vi "Read Anything.vi"(7 "Type of Anything":variant, 8 "Error In":errorcluster, 9 "Section Name (Name of \"Type of Anything\")":string, 11 "Path (dialog)":path) -> (0 "Error Out":errorcluster, 1 "Found?":bool, 3 "Anything":variant)   [LabVIEW 2012]
doc: "This VI is designed to read data from a file written by <B>Write Anything.vi</B>. If the data type definition has changed since it was written to file, this VI will still read and fill out any elements of the cluster that have the same name. Any elements for which it cannot find a name match in the file will be supplied with their datatype's default value.\n\nFreeware from Moore Good Ideas, www.mooregoodideas.com. Do not remove this line."
uses:
  <vilib>/Utility/VariantDataType/VariantType.lvlib
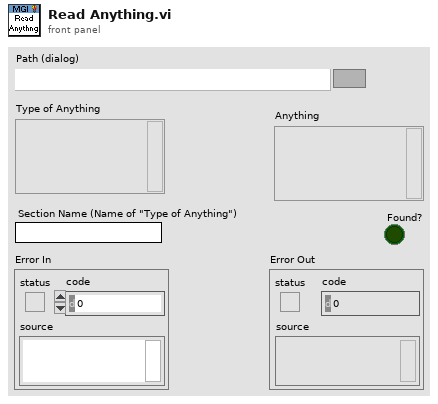
[diagram p1: front panel]
types:
  T1 = typedef "VariantType.lvlib/Type.ctl" = enum8{"Invalid Type", "Void", "I8", "I16", "I32", "I64", "U8", "U16", "U32", "U64", "Single Float", "Double Float", "Extended Float", "Single Complex", "Double Complex", "Extended Complex", "Enum U8", "Enum U16", "Enum U32", "Enum U64", "Single Float With Unit", "Double Float With Unit", "Extended Float With Unit", "Single Complex with Unit", "Double Complex with Unit", "Extended Complex with Unit", "Boolean", "String", "Path", "Picture", "Tag", "Array", "Cluster", "Variant", "LV Variant", "Waveform", "Timestamp", "Digital Waveform", "Digital Data", "ExpressData", "Refnum", "External Data", "VI", "Poly VI", "LabVIEW Class Instance", "Fixed Point"}
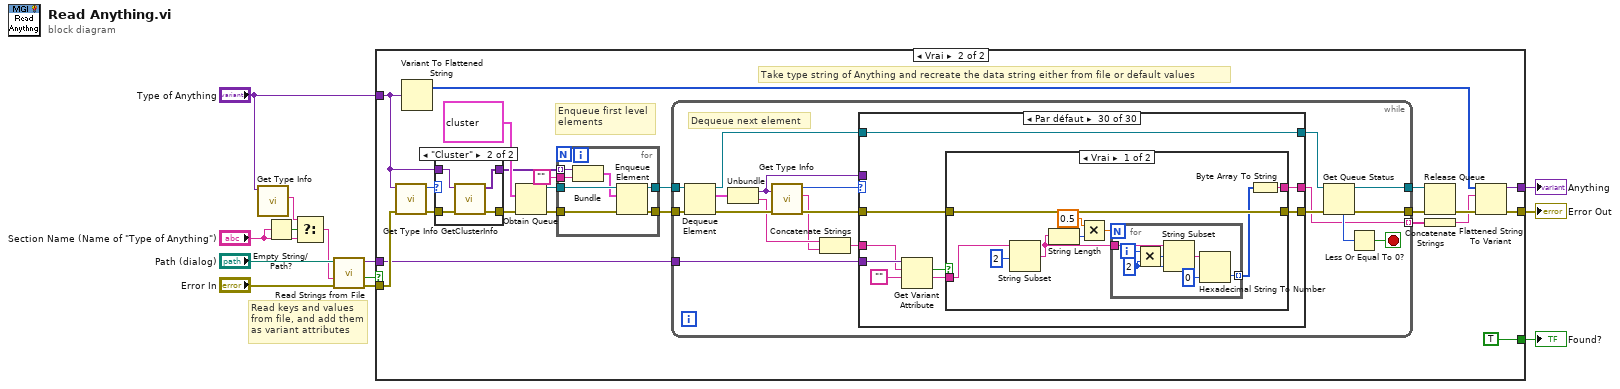
[diagram p0: block diagram]
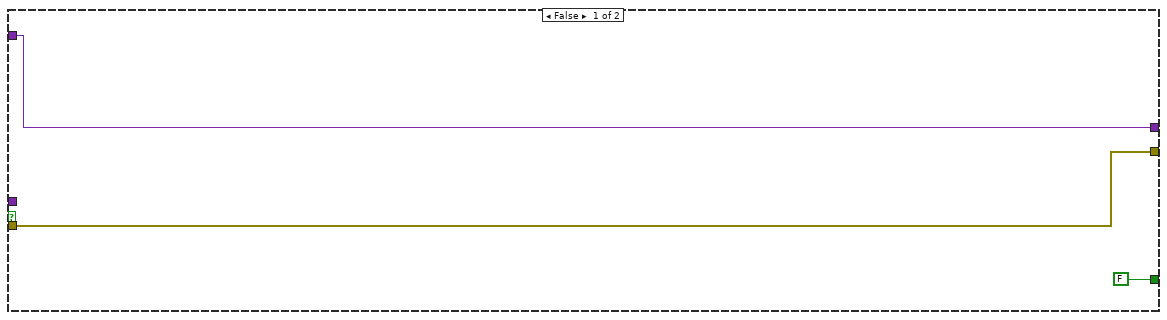
[diagram p2: hidden frame]
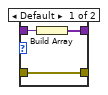
[diagram p3: hidden frame]
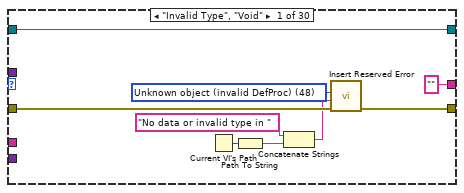
[diagram p4: hidden frame]
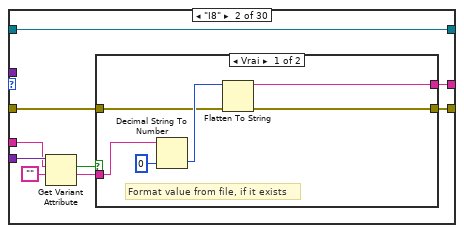
[diagram p5: hidden frame]
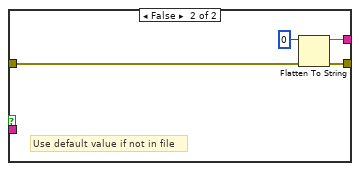
[diagram p6: hidden frame]
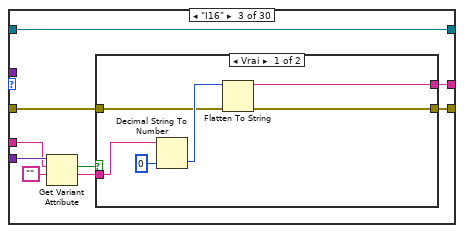
[diagram p7: hidden frame]
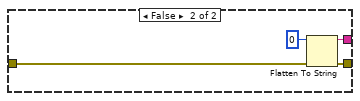
[diagram p8: hidden frame]
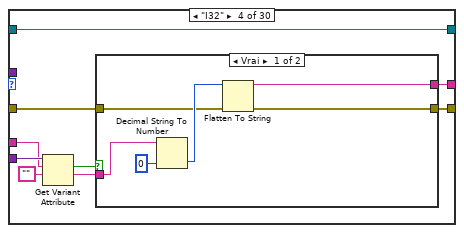
[diagram p9: hidden frame]
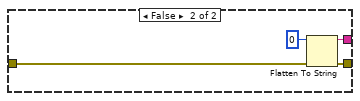
[diagram p10: hidden frame]
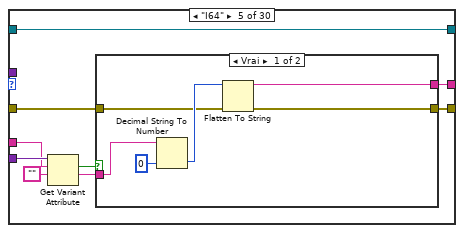
[diagram p11: hidden frame]
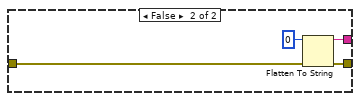
[diagram p12: hidden frame]
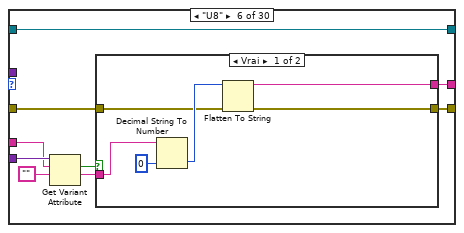
[diagram p13: hidden frame]
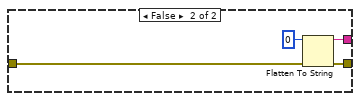
[diagram p14: hidden frame]
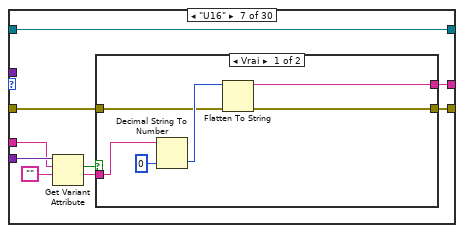
[diagram p15: hidden frame]
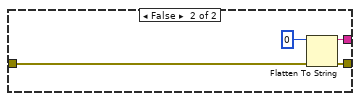
[diagram p16: hidden frame]
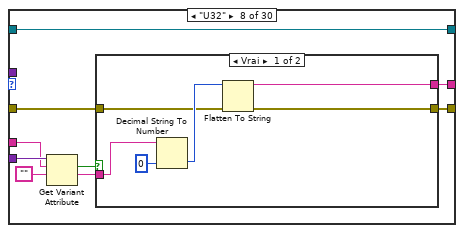
[diagram p17: hidden frame]
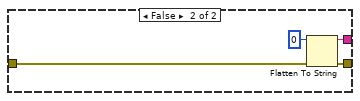
[diagram p18: hidden frame]
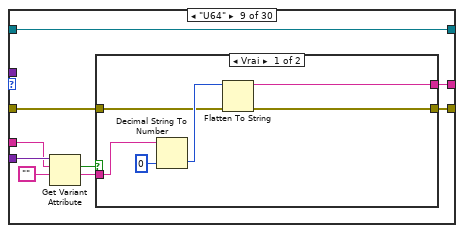
[diagram p19: hidden frame]
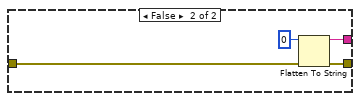
[diagram p20: hidden frame]
diagram:
  # "Read keys and values from file, and add them as variant attributes"
  n1 = call "Get Type Info.vi"("Variant"="Type of Anything") -> ("Name"=w2:string)  [unwired: 8 in, 2 out]
  n2 = Empty String/Path?(string/path="Section Name (Name of \"Type of Anything\")") -> (empty?=w5:bool)
  n3 = Select(t=w2, s=w5, f="Section Name (Name of \"Type of Anything\")") -> (s? t:f=w3:string)
  n4 = call "Read Strings from File.vi"("Error In"="Error In", "Section Name"=w3, "Path"="Path (dialog)") -> ("Error Out"=w11:errorcluster, "Found?"=w8:bool, "Variant Database"=w7:variant)  [unwired: 6 in]
  n5 = case shown="Vrai" w8 {
    tunnel: [w15 w37] -> w13
    tunnel: [w16 w36] -> w12
    tunnel: "Type of Anything" -> [w16 w18]
    tunnel: w11 -> [w15 w24]
    tunnel: [FALSE TRUE] -> w9
    tunnel: w7 -> [_ w22]
    frame False {
    }
    frame True {
      # "Enqueue first level\nelements"
      # "Take type string of Anything and recreate the data string either from file or default values"
      n6 = call "Get Type Info.vi"("Error In"=w24, "Variant"=w18) -> ("Error Out"=w19:errorcluster, "Type Enum"=w21:T1)  [unwired: 7 in, 1 out]
      n7 = Variant To Flattened String(Variant=w18) -> (1:w38:i16[])  [unwired: 1 out]
      n8 = case shown="\"Cluster\"" w21 {
        tunnel: [w41 w44] -> w20
        tunnel: w19 -> [w41 w45]
        tunnel: w18 -> [w40 w43]
        tunnel: [w39 w42] -> w17
        frame Default {
          n9 = Build Array(w40) -> (w39:variant[])
        }
        frame "Cluster" {
          n10 = call <vilib>:"GetClusterInfo.vi"("error in (no error)"=w45, "Variant"=w43) -> ("error out"=w44:errorcluster, "Cluster Elements"=w42:variant[])  [unwired: 8 in]
        }
      }
      n11 = Obtain Queue(element data type=cluster{"Variant":variant, "Name":string} {"Variant"=variant, "Name"=""}, error in (no error)=w20) -> (queue out=w34:refnum<queue>, error out=w26:errorcluster)  [unwired: 3 in, 1 out]
      n12 = for {
        tunnel: w34 -> [w52]
        tunnel: [w51] -> w33
        tunnel: [w50] -> w32
        tunnel: w17 -> [w49] mode=indexing
        tunnel: "" -> [w47]
        tunnel: w26 -> [w46]
        n13 = Bundle("ArrayElt"=w49, w47) -> (w48:cluster{"ArrayElt":variant, string})  [unwired: 1 in]
        n14 = Enqueue Element(queue=w52, element=w48, error in (no error)=w46) -> (queue out=w50:refnum<queue>, error out=w51:errorcluster)  [unwired: 1 in, 1 out]
      }
      n15 = while {
        tunnel: w33 -> [w69]
        tunnel: [w64] -> w31
        tunnel: w22 -> [w56]
        tunnel: [w53] -> w35 mode=indexing
        tunnel: w32 -> [w66]
        tunnel: [w60] -> w29
        stop <- w61 stop-if-true
        # "Dequeue next element"
        n16 = Dequeue Element(queue=w66, error in (no error)=w69) -> (queue out=w67:refnum<queue>, element=w59:cluster{"Variant":variant, "Name":string}, error out=w68:errorcluster)  [unwired: 1 in, 1 out]
        n17 = Unbundle(w59) -> ("Variant"=w55:variant, "Name"=w57:string)
        n18 = call "Get Type Info.vi"("Error In"=w68, "Variant"=w55) -> ("Error Out"=w70:errorcluster, "Name"=w54:string, "Type Enum"=w71:T1)  [unwired: 7 in]
        n19 = Concatenate Strings(w57, w54) -> (w58:string)
        n20 = case shown="Par défaut" w71 {
          tunnel: [w74 w89 w108 w127 w146 w165 w184 w203 w222 w241 w261 w281 w301 w320 w339 w359 w385 w411 w437 w462 w481 w498 w513 w535 w564 w593 w622 w651 w679 w691] -> w65
          tunnel: w70 -> [w75 w88 w107 w126 w145 w164 w183 w202 w221 w240 w260 w280 w300 w319 w338 w358 w384 w410 w436 w461 w480 w497 w519 w534 w563 w592 w621 w650 w680 w690]
          tunnel: w58 -> [_ w83 w102 w121 w140 w159 w177 w197 w216 w235 w254 w275 w294 w314 w334 w351 w377 w404 w430 w456 w475 w491 w509 w529 w558 w586 w614 w644 w674 w683]
          tunnel: ["" ("data string") w87 w106 w125 w144 w163 w182 w201 w220 w239 w259 w279 w299 w318 w337 w357 w383 w409 w435 w460 w479 w496 "" w533 w562 w591 w620 w649 w677 w689] -> w53
          tunnel: w55 -> [_ _ _ _ _ _ _ _ _ _ _ _ _ _ _ w356 w382 w408 w434 _ _ _ w518 _ _ _ _ _ w678 _]
          tunnel: w67 -> [w76 w86 w105 w124 w143 w162 w181 w200 w219 w238 w258 w278 w298 w317 w336 w355 w381 w407 w433 w459 w478 w495 w514 w532 w561 w590 w619 w648 w682 w688]
          tunnel: [w76 w86 w105 w124 w143 w162 w181 w200 w219 w238 w258 w278 w298 w317 w336 w355 w381 w407 w433 w459 w478 w495 w512 w532 w561 w590 w619 w648 w681 w688] -> w63
          tunnel: w56 -> [_ w84 w103 w122 w141 w160 w178 w198 w217 w237 w255 w276 w295 w315 w335 w353 w378 w405 w431 w457 w476 w492 _ w530 w559 w588 w617 w645 w675 w686]
          frame "Invalid Type", "Void" {
            w72 = u16 48 items=["No error", "Argument error", "Memory is full", "Out of zone", "End of file", "File already open", "Generic file I/O error", "File not found", "File permission error", "Disk is full", "Duplicate path", "Too many files open", "System feature not enabled", "Resource file not found", "Cannot add resource", "Resource not found", "Image not found", "Image memory error", "Pen does not exist", "Config type invalid", "Config token not found", "Config parse error", "Config memory error", "Bad external code format", "Bad external code offset", "External code not present", "Null window", "Destroy window error", "Null menu", "Print aborted", "Bad print record", "Print driver error", "Windows error during printing", "Memory error during printing", "Print dialog error", "Generic print error", "Invalid device refnum", "Device not found", "Device parameter error", "Device unit error", "Cannot open device", "Device call aborted", "Generic error", "Cancelled by user", "Object ID too low", "Object ID too high", "Object not in heap", "Unknown heap", "Unknown object (invalid DefProc)", "Unknown object (DefProc not in table)", "Message out of range", "Invalid (null) method", "Unknown message", "Manager call not supported", "Bad address", "Network operation in progress", "Network operation timed out", "Connection is busy", "Network attribute not supported", "Network error", "Address in use", "System out of memory", "Connection aborted", "Connection refused", "Not connected", "Already connected", "Connection closed", "Initialization error (interapplication manager)", "Bad occurrence", "Wait on unbound occurrence handler", "Occurrence queue overflow", "Datalog type conflict", "Unused", "Unrecognized type (interapplication manager)", "Memory corrupt", "Failed to make temporary DLL", "Old CIN version", "Drag socket not found", "Failed to load drop-object", "Failed to register OLE object", "Failed to release OLE object", "Format specifier type mismatch", "Unknown format specifier", "Too few format specifiers", "Too many format specifiers", "Scan failed", "Newer CIN version", "OLE Convert", "Runtime menu error", "Password tampered", "Unknown error code"] ("Reserved Error Code")
            n21 = Current VI's Path() -> (path=w78:path)
            n22 = Path To String(path=w78) -> (string=w77:string)
            n23 = Concatenate Strings("No data or invalid type in " ("string"), w77) -> (w73:string)
            n24 = call "Insert Reserved Error.vi"("error in (no error)"=w75, "non-standard source (\"\")"=w73, "Reserved Error Code"=w72) -> ("error out"=w74:errorcluster)  [unwired: 4 in]
          }
          frame "I8" {
            n25 = Get Variant Attribute(Variant=w84, name=w83, default value (empty Variant)="") -> (found=w81:bool, value=w82:string)  [unwired: 1 in, 2 out]
            n26 = case shown="Vrai" w81 {
              tunnel: w82 -> [w90 _]
              tunnel: [w93 w96] -> w89
              tunnel: w88 -> [w92 w97]
              tunnel: [w94 w99] -> w87
              frame True {
                # "Format value from file, if it exists"
                n27 = Decimal String To Number(string=w90, default (0L)=i8 0 ("default (0 I32)")) -> (number=w95:i8)  [unwired: 1 in, 1 out]
                n28 = Flatten To String(anything=w95, error in (no error)=w92) -> (data string=w94:string, error out=w93:errorcluster)  [unwired: 2 in, 1 out]
              }
              frame False {
                # "Use default value if not in file"
                n29 = Flatten To String(anything=i8 0, error in (no error)=w97) -> (data string=w99:string, error out=w96:errorcluster)  [unwired: 2 in, 1 out]
              }
            }
          }
          frame "I16" {
            n30 = Get Variant Attribute(Variant=w103, name=w102, default value (empty Variant)="") -> (found=w100:bool, value=w101:string)  [unwired: 1 in, 2 out]
            n31 = case shown="Vrai" w100 {
              tunnel: w101 -> [w109 _]
              tunnel: [w112 w115] -> w108
              tunnel: w107 -> [w111 w116]
              tunnel: [w113 w118] -> w106
              frame True {
                n32 = Decimal String To Number(string=w109, default (0L)=i16 0 ("default (0 I32)")) -> (number=w114:i16)  [unwired: 1 in, 1 out]
                n33 = Flatten To String(anything=w114, error in (no error)=w111) -> (data string=w113:string, error out=w112:errorcluster)  [unwired: 2 in, 1 out]
              }
              frame False {
                n34 = Flatten To String(anything=i16 0, error in (no error)=w116) -> (data string=w118:string, error out=w115:errorcluster)  [unwired: 2 in, 1 out]
              }
            }
          }
          frame "I32" {
            n35 = Get Variant Attribute(Variant=w122, name=w121, default value (empty Variant)="") -> (found=w119:bool, value=w120:string)  [unwired: 1 in, 2 out]
            n36 = case shown="Vrai" w119 {
              tunnel: w120 -> [w128 _]
              tunnel: [w131 w134] -> w127
              tunnel: w126 -> [w130 w135]
              tunnel: [w132 w137] -> w125
              frame True {
                n37 = Decimal String To Number(string=w128, default (0L)=0 ("default (0 I32)")) -> (number=w133:i32)  [unwired: 1 in, 1 out]
                n38 = Flatten To String(anything=w133, error in (no error)=w130) -> (data string=w132:string, error out=w131:errorcluster)  [unwired: 2 in, 1 out]
              }
              frame False {
                n39 = Flatten To String(anything=0, error in (no error)=w135) -> (data string=w137:string, error out=w134:errorcluster)  [unwired: 2 in, 1 out]
              }
            }
          }
          frame "I64" {
            n40 = Get Variant Attribute(Variant=w141, name=w140, default value (empty Variant)="") -> (found=w138:bool, value=w139:string)  [unwired: 1 in, 2 out]
            n41 = case shown="Vrai" w138 {
              tunnel: w139 -> [w147 _]
              tunnel: [w150 w153] -> w146
              tunnel: w145 -> [w149 w154]
              tunnel: [w151 w156] -> w144
              frame True {
                n42 = Decimal String To Number(string=w147, default (0L)=i64 0 ("default (0 I32)")) -> (number=w152:i64)  [unwired: 1 in, 1 out]
                n43 = Flatten To String(anything=w152, error in (no error)=w149) -> (data string=w151:string, error out=w150:errorcluster)  [unwired: 2 in, 1 out]
              }
              frame False {
                n44 = Flatten To String(anything=i64 0, error in (no error)=w154) -> (data string=w156:string, error out=w153:errorcluster)  [unwired: 2 in, 1 out]
              }
            }
          }
          frame "U8" {
            n45 = Get Variant Attribute(Variant=w160, name=w159, default value (empty Variant)="") -> (found=w157:bool, value=w158:string)  [unwired: 1 in, 2 out]
            n46 = case shown="Vrai" w157 {
              tunnel: w158 -> [w166 _]
              tunnel: [w169 w172] -> w165
              tunnel: w164 -> [w168 w173]
              tunnel: [w170 w175] -> w163
              frame True {
                n47 = Decimal String To Number(string=w166, default (0L)=u8 0 ("default (0 I32)")) -> (number=w171:u8)  [unwired: 1 in, 1 out]
                n48 = Flatten To String(anything=w171, error in (no error)=w168) -> (data string=w170:string, error out=w169:errorcluster)  [unwired: 2 in, 1 out]
              }
              frame False {
                n49 = Flatten To String(anything=u8 0, error in (no error)=w173) -> (data string=w175:string, error out=w172:errorcluster)  [unwired: 2 in, 1 out]
              }
            }
          }
          frame "U16" {
            n50 = Get Variant Attribute(Variant=w178, name=w177, default value (empty Variant)="") -> (found=w176:bool, value=w179:string)  [unwired: 1 in, 2 out]
            n51 = case shown="Vrai" w176 {
              tunnel: w179 -> [w185 _]
              tunnel: [w188 w191] -> w184
              tunnel: w183 -> [w187 w192]
              tunnel: [w189 w194] -> w182
              frame True {
                n52 = Decimal String To Number(string=w185, default (0L)=u16 0 ("default (0 I32)")) -> (number=w190:u16)  [unwired: 1 in, 1 out]
                n53 = Flatten To String(anything=w190, error in (no error)=w187) -> (data string=w189:string, error out=w188:errorcluster)  [unwired: 2 in, 1 out]
              }
              frame False {
                n54 = Flatten To String(anything=u16 0, error in (no error)=w192) -> (data string=w194:string, error out=w191:errorcluster)  [unwired: 2 in, 1 out]
              }
            }
          }
          frame "U32" {
            n55 = Get Variant Attribute(Variant=w198, name=w197, default value (empty Variant)="") -> (found=w195:bool, value=w196:string)  [unwired: 1 in, 2 out]
            n56 = case shown="Vrai" w195 {
              tunnel: w196 -> [w204 _]
              tunnel: [w207 w210] -> w203
              tunnel: w202 -> [w206 w211]
              tunnel: [w208 w213] -> w201
              frame True {
                n57 = Decimal String To Number(string=w204, default (0L)=u32 0 ("default (0 I32)")) -> (number=w209:u32)  [unwired: 1 in, 1 out]
                n58 = Flatten To String(anything=w209, error in (no error)=w206) -> (data string=w208:string, error out=w207:errorcluster)  [unwired: 2 in, 1 out]
              }
              frame False {
                n59 = Flatten To String(anything=u32 0, error in (no error)=w211) -> (data string=w213:string, error out=w210:errorcluster)  [unwired: 2 in, 1 out]
              }
            }
          }
          frame "U64" {
            n60 = Get Variant Attribute(Variant=w217, name=w216, default value (empty Variant)="") -> (found=w214:bool, value=w215:string)  [unwired: 1 in, 2 out]
            n61 = case shown="Vrai" w214 {
              tunnel: w215 -> [w223 _]
              tunnel: [w226 w229] -> w222
              tunnel: w221 -> [w225 w230]
              tunnel: [w227 w232] -> w220
              frame True {
                n62 = Decimal String To Number(string=w223, default (0L)=u64 0 ("default (0 I32)")) -> (number=w228:u64)  [unwired: 1 in, 1 out]
                n63 = Flatten To String(anything=w228, error in (no error)=w225) -> (data string=w227:string, error out=w226:errorcluster)  [unwired: 2 in, 1 out]
              }
              frame False {
                n64 = Flatten To String(anything=u64 0, error in (no error)=w230) -> (data string=w232:string, error out=w229:errorcluster)  [unwired: 2 in, 1 out]
              }
            }
          }
          frame "Single Float", "Single Float With Unit" {
            n65 = Get Variant Attribute(Variant=w237, name=w235, default value (empty Variant)="") -> (found=w233:bool, value=w234:string)  [unwired: 1 in, 2 out]
            n66 = case shown="Vrai" w233 {
              tunnel: w234 -> [w243 _]
              tunnel: [w246 w249] -> w241
              tunnel: w240 -> [w245 w250]
              tunnel: [w247 w252] -> w239
              frame True {
                n67 = Fract/Exp String To Number(use system decimal point (T)=FALSE ("utiliser le séparateur décimal du système (V)"), string=w243, default (0 dbl)=sgl 0.0 ("default (0 I32)")) -> (number=w248:sgl)  [unwired: 1 in, 1 out]
                n68 = Flatten To String(anything=w248, error in (no error)=w245) -> (data string=w247:string, error out=w246:errorcluster)  [unwired: 2 in, 1 out]
              }
              frame False {
                n69 = Flatten To String(anything=sgl 0.0, error in (no error)=w250) -> (data string=w252:string, error out=w249:errorcluster)  [unwired: 2 in, 1 out]
              }
            }
          }
          frame "Double Float", "Double Float With Unit" {
            n70 = Get Variant Attribute(Variant=w255, name=w254, default value (empty Variant)="") -> (found=w253:bool, value=w256:string)  [unwired: 1 in, 2 out]
            n71 = case shown="Vrai" w253 {
              tunnel: w256 -> [w263 _]
              tunnel: [w266 w269] -> w261
              tunnel: w260 -> [w265 w270]
              tunnel: [w267 w272] -> w259
              frame True {
                n72 = Fract/Exp String To Number(use system decimal point (T)=FALSE ("utiliser le séparateur décimal du système (V)"), string=w263, default (0 dbl)=0.0 ("default (0 DBL)")) -> (number=w268:dbl)  [unwired: 1 in, 1 out]
                n73 = Flatten To String(anything=w268, error in (no error)=w265) -> (data string=w267:string, error out=w266:errorcluster)  [unwired: 2 in, 1 out]
              }
              frame False {
                n74 = Flatten To String(anything=0.0, error in (no error)=w270) -> (data string=w272:string, error out=w269:errorcluster)  [unwired: 2 in, 1 out]
              }
            }
          }
          frame "Extended Float", "Extended Float With Unit" {
            n75 = Get Variant Attribute(Variant=w276, name=w275, default value (empty Variant)="") -> (found=w273:bool, value=w274:string)  [unwired: 1 in, 2 out]
            n76 = case shown="Vrai" w273 {
              tunnel: w274 -> [w283 _]
              tunnel: [w286 w289] -> w281
              tunnel: w280 -> [w285 w290]
              tunnel: [w287 w292] -> w279
              frame True {
                n77 = Fract/Exp String To Number(use system decimal point (T)=FALSE ("utiliser le séparateur décimal du système (V)"), string=w283, default (0 dbl)=ext 0.0 ("default (0 DBL)")) -> (number=w288:ext)  [unwired: 1 in, 1 out]
                n78 = Flatten To String(anything=w288, error in (no error)=w285) -> (data string=w287:string, error out=w286:errorcluster)  [unwired: 2 in, 1 out]
              }
              frame False {
                n79 = Flatten To String(anything=ext 0.0, error in (no error)=w290) -> (data string=w292:string, error out=w289:errorcluster)  [unwired: 2 in, 1 out]
              }
            }
          }
          frame "Single Complex", "Single Complex with Unit" {
            n80 = Get Variant Attribute(Variant=w295, name=w294, default value (empty Variant)="") -> (found=w293:bool, value=w296:string)  [unwired: 1 in, 2 out]
            n81 = case shown="Vrai" w293 {
              tunnel: w296 -> [w302 _]
              tunnel: [w306 w308] -> w301
              tunnel: w300 -> [w305 w309]
              tunnel: [w307 w311] -> w299
              frame True {
                n82 = Scan From String(input string=w302, default 1=csg 0.0+0.0i ("default (0 DBL)")) -> (output 1=w303:csg)  [unwired: 3 in, 3 out]
                n83 = Flatten To String(anything=w303, error in (no error)=w305) -> (data string=w307:string, error out=w306:errorcluster)  [unwired: 2 in, 1 out]
              }
              frame False {
                n84 = Flatten To String(anything=csg 0.0+0.0i, error in (no error)=w309) -> (data string=w311:string, error out=w308:errorcluster)  [unwired: 2 in, 1 out]
              }
            }
          }
          frame "Double Complex", "Double Complex with Unit" {
            n85 = Get Variant Attribute(Variant=w315, name=w314, default value (empty Variant)="") -> (found=w312:bool, value=w313:string)  [unwired: 1 in, 2 out]
            n86 = case shown="Vrai" w312 {
              tunnel: w313 -> [w321 _]
              tunnel: [w325 w327] -> w320
              tunnel: w319 -> [w324 w328]
              tunnel: [w326 w330] -> w318
              frame True {
                n87 = Scan From String(input string=w321, default 1=cdb 0.0+0.0i ("default (0 DBL)")) -> (output 1=w323:cdb)  [unwired: 3 in, 3 out]
                n88 = Flatten To String(anything=w323, error in (no error)=w324) -> (data string=w326:string, error out=w325:errorcluster)  [unwired: 2 in, 1 out]
              }
              frame False {
                n89 = Flatten To String(anything=cdb 0.0+0.0i, error in (no error)=w328) -> (data string=w330:string, error out=w327:errorcluster)  [unwired: 2 in, 1 out]
              }
            }
          }
          frame "Extended Complex", "Extended Complex with Unit" {
            n90 = Get Variant Attribute(Variant=w335, name=w334, default value (empty Variant)="") -> (found=w331:bool, value=w332:string)  [unwired: 1 in, 2 out]
            n91 = case shown="Vrai" w331 {
              tunnel: w332 -> [w340 _]
              tunnel: [w344 w346] -> w339
              tunnel: w338 -> [w343 w347]
              tunnel: [w345 w349] -> w337
              frame True {
                n92 = Scan From String(input string=w340, default 1=cxt 0.0+0.0i ("default (0 DBL)")) -> (output 1=w341:cxt)  [unwired: 3 in, 3 out]
                n93 = Flatten To String(anything=w341, error in (no error)=w343) -> (data string=w345:string, error out=w344:errorcluster)  [unwired: 2 in, 1 out]
              }
              frame False {
                n94 = Flatten To String(anything=cxt 0.0+0.0i, error in (no error)=w347) -> (data string=w349:string, error out=w346:errorcluster)  [unwired: 2 in, 1 out]
              }
            }
          }
          frame "Enum U8" {
            n95 = Get Variant Attribute(Variant=w353, name=w351, default value (empty Variant)="") -> (found=w350:bool, value=w352:string)  [unwired: 1 in, 2 out]
            n96 = case shown="Vrai" w350 {
              tunnel: w352 -> [w360 _]
              tunnel: [w370 w373] -> w359
              tunnel: w358 -> [w369 w374]
              tunnel: [w371 w375] -> w357
              tunnel: w356 -> [w368 _]
              frame True {
                n97 = call <vilib>:"GetNumericInfo.vi"("error in (no error)"=w369, "Variant"=w368) -> ("error out"=w361:errorcluster, "EnumNames"=w367:string[])  [unwired: 6 in, 2 out]
                n98 = Search 1D Array(1D array=w367, element=w360) -> (index of element=w366:i32)  [unwired: 1 in]
                n99 = In Range and Coerce(upper limit=255, x=w366, lower limit=0) -> (coerced(x)=w364:i32)  [unwired: 1 out]
                n100 = To Unsigned Byte Integer(number=w364) -> (unsigned 8bit integer=w365:u8)
                n101 = Flatten To String(anything=w365, error in (no error)=w361) -> (data string=w371:string, error out=w370:errorcluster)  [unwired: 2 in, 1 out]
              }
              frame False {
                n102 = Flatten To String(anything=u8 0, error in (no error)=w374) -> (data string=w375:string, error out=w373:errorcluster)  [unwired: 2 in, 1 out]
              }
            }
          }
          frame "Enum U16" {
            n103 = Get Variant Attribute(Variant=w378, name=w377, default value (empty Variant)="") -> (found=w376:bool, value=w379:string)  [unwired: 1 in, 2 out]
            n104 = case shown="Vrai" w376 {
              tunnel: w379 -> [w386 _]
              tunnel: [w396 w399] -> w385
              tunnel: w384 -> [w395 w400]
              tunnel: [w397 w401] -> w383
              tunnel: w382 -> [w394 _]
              frame True {
                n105 = call <vilib>:"GetNumericInfo.vi"("error in (no error)"=w395, "Variant"=w394) -> ("error out"=w387:errorcluster, "EnumNames"=w393:string[])  [unwired: 6 in, 2 out]
                n106 = Search 1D Array(1D array=w393, element=w386) -> (index of element=w392:i32)  [unwired: 1 in]
                n107 = In Range and Coerce(upper limit=u16 65535, x=w392, lower limit=0) -> (coerced(x)=w390:i32)  [unwired: 1 out]
                n108 = To Unsigned Word Integer(number=w390) -> (unsigned 16bit integer=w391:u16)
                n109 = Flatten To String(anything=w391, error in (no error)=w387) -> (data string=w397:string, error out=w396:errorcluster)  [unwired: 2 in, 1 out]
              }
              frame False {
                n110 = Flatten To String(anything=u16 0, error in (no error)=w400) -> (data string=w401:string, error out=w399:errorcluster)  [unwired: 2 in, 1 out]
              }
            }
          }
          frame "Enum U32" {
            n111 = Get Variant Attribute(Variant=w405, name=w404, default value (empty Variant)="") -> (found=w402:bool, value=w403:string)  [unwired: 1 in, 2 out]
            n112 = case shown="Vrai" w402 {
              tunnel: w403 -> [w412 _]
              tunnel: [w422 w425] -> w411
              tunnel: w410 -> [w421 w426]
              tunnel: [w423 w427] -> w409
              tunnel: w408 -> [w420 _]
              frame True {
                n113 = call <vilib>:"GetNumericInfo.vi"("error in (no error)"=w421, "Variant"=w420) -> ("error out"=w413:errorcluster, "EnumNames"=w419:string[])  [unwired: 6 in, 2 out]
                n114 = Search 1D Array(1D array=w419, element=w412) -> (index of element=w418:i32)  [unwired: 1 in]
                n115 = In Range and Coerce(upper limit=u32 4294967295, x=w418, lower limit=0) -> (coerced(x)=w416:u32)  [unwired: 1 out]
                n116 = To Unsigned Long Integer(number=w416) -> (unsigned 32bit integer=w417:u32)
                n117 = Flatten To String(anything=w417, error in (no error)=w413) -> (data string=w423:string, error out=w422:errorcluster)  [unwired: 2 in, 1 out]
              }
              frame False {
                n118 = Flatten To String(anything=u32 0, error in (no error)=w426) -> (data string=w427:string, error out=w425:errorcluster)  [unwired: 2 in, 1 out]
              }
            }
          }
          frame "Enum U64" {
            n119 = Get Variant Attribute(Variant=w431, name=w430, default value (empty Variant)="") -> (found=w428:bool, value=w429:string)  [unwired: 1 in, 2 out]
            n120 = case shown="Vrai" w428 {
              tunnel: [w448 w451] -> w437
              tunnel: w436 -> [w447 w452]
              tunnel: [w449 w453] -> w435
              tunnel: w434 -> [w446 _]
              tunnel: w429 -> [w438 _]
              frame True {
                n121 = call <vilib>:"GetNumericInfo.vi"("error in (no error)"=w447, "Variant"=w446) -> ("error out"=w439:errorcluster, "EnumNames"=w445:string[])  [unwired: 6 in, 2 out]
                n122 = Search 1D Array(1D array=w445, element=w438) -> (index of element=w444:i32)  [unwired: 1 in]
                n123 = In Range and Coerce(upper limit=u64 18446744073709551615, x=w444, lower limit=0) -> (coerced(x)=w442:u64)  [unwired: 1 out]
                n124 = To Unsigned Quad Integer(1:w442) -> (0:w443:u64)
                n125 = Flatten To String(anything=w443, error in (no error)=w439) -> (data string=w449:string, error out=w448:errorcluster)  [unwired: 2 in, 1 out]
              }
              frame False {
                n126 = Flatten To String(anything=u64 0, error in (no error)=w452) -> (data string=w453:string, error out=w451:errorcluster)  [unwired: 2 in, 1 out]
              }
            }
          }
          frame "Boolean" {
            n127 = Get Variant Attribute(Variant=w457, name=w456, default value (empty Variant)="") -> (found=w454:bool, value=w455:string)  [unwired: 1 in, 2 out]
            n128 = case shown="Vrai" w454 {
              tunnel: w455 -> [w463 _]
              tunnel: [w467 w470] -> w462
              tunnel: w461 -> [w464 w471]
              tunnel: [w468 w472] -> w460
              frame True {
                n129 = Equal?(x=w463, y="TRUE") -> (x = y?=w465:bool)
                n130 = Flatten To String(anything=w465, error in (no error)=w464) -> (data string=w468:string, error out=w467:errorcluster)  [unwired: 2 in, 1 out]
              }
              frame False {
                n131 = Flatten To String(anything=FALSE, error in (no error)=w471) -> (data string=w472:string, error out=w470:errorcluster)  [unwired: 2 in, 1 out]
              }
            }
          }
          frame "String" {
            n132 = Get Variant Attribute(Variant=w476, name=w475, default value (empty Variant)="") -> (found=w474:bool, value=w473:string)  [unwired: 1 in, 2 out]
            n133 = case shown="Vrai" w474 {
              tunnel: [w484 w487] -> w481
              tunnel: w480 -> [w483 w488]
              tunnel: [w485 w489] -> w479
              tunnel: w473 -> [w482 _]
              frame True {
                n134 = Flatten To String(anything=w482, error in (no error)=w483) -> (data string=w485:string, error out=w484:errorcluster)  [unwired: 2 in, 1 out]
              }
              frame False {
                n135 = Flatten To String(anything="", error in (no error)=w488) -> (data string=w489:string, error out=w487:errorcluster)  [unwired: 2 in, 1 out]
              }
            }
          }
          frame "Path" {
            n136 = Get Variant Attribute(Variant=w492, name=w491, default value (empty Variant)="") -> (found=w493:bool, value=w490:string)  [unwired: 1 in, 2 out]
            n137 = case shown="Vrai" w493 {
              tunnel: [w502 w505] -> w498
              tunnel: w497 -> [w501 w506]
              tunnel: [w503 w507] -> w496
              tunnel: w490 -> [w499 _]
              frame True {
                n138 = String To Path(string=w499) -> (path=w500:path)
                n139 = Flatten To String(anything=w500, error in (no error)=w501) -> (data string=w503:string, error out=w502:errorcluster)  [unwired: 2 in, 1 out]
              }
              frame False {
                n140 = Flatten To String(anything=path "", error in (no error)=w506) -> (data string=w507:string, error out=w505:errorcluster)  [unwired: 2 in, 1 out]
              }
            }
          }
          frame "Cluster" {
            # "Enqueue cluster elements"
            n141 = call <vilib>:"GetClusterInfo.vi"("error in (no error)"=w519, "Variant"=w518) -> ("error out"=w515:errorcluster, "Cluster Elements"=w517:variant[])  [unwired: 8 in]
            n142 = Concatenate Strings(w509, "." ("string")) -> (w508:string)
            n143 = Reverse 1D Array(array=w517) -> (reversed array=w516:variant[])
            n144 = for {
              tunnel: w514 -> [w526]
              tunnel: w515 -> [w525]
              tunnel: [w524] -> w513
              tunnel: [w523] -> w512
              tunnel: w516 -> [w522] mode=indexing
              tunnel: w508 -> [w520]
              n145 = Bundle("ArrayElt"=w522, w520) -> (w521:cluster{"ArrayElt":variant, string})  [unwired: 1 in]
              n146 = Enqueue Element At Opposite End(queue=w526, element=w521, error in (no error)=w525) -> (queue out=w523:refnum<queue>, error out=w524:errorcluster)  [unwired: 1 in, 1 out]
            }
          }
          frame "Variant", "LV Variant" {
            n147 = Get Variant Attribute(Variant=w530, name=w529, default value (empty Variant)="") -> (found=w527:bool, value=w528:string)  [unwired: 1 in, 2 out]
            n148 = case shown="Vrai" w527 {
              tunnel: w528 -> [w536 _]
              tunnel: [w544 w553] -> w535
              tunnel: w534 -> [w544 w554]
              tunnel: [w542 w555] -> w533
              frame True {
                n149 = String Subset(string=w536, offset (0)=2) -> (substring=w541:string)  [unwired: 1 in]
                n150 = String Length(string=w541) -> (length=w539:i32)
                n151 = Multiply(x=0.5, y=w539) -> (x*y=w538:dbl)
                n152 = for {
                  N: w538 -> [_]
                  tunnel: w541 -> [w548]
                  tunnel: [w550] -> w540 mode=indexing
                  i -> [w547]
                  w546 = 2 ("length (rest)")
                  n153 = Multiply(x=w547, y=w546) -> (x*y=w545:i32)
                  n154 = String Subset(string=w548, offset (0)=w545, length (rest)=w546) -> (substring=w549:string)
                  n155 = Hexadecimal String To Number(string=w549, default (0uL)=u8 0 ("default (0 U32)")) -> (number=w550:u8)  [unwired: 1 in, 1 out]
                }
                n156 = Byte Array To String(unsigned byte array=w540) -> (string=w542:string)
              }
              frame False {
                w552 = variant  # Variant
                n157 = Flatten To String(anything=w552, error in (no error)=w554) -> (data string=w555:string, error out=w553:errorcluster)  [unwired: 2 in, 1 out]
              }
            }
          }
          frame "Waveform" {
            n158 = Get Variant Attribute(Variant=w559, name=w558, default value (empty Variant)="") -> (found=w556:bool, value=w557:string)  [unwired: 1 in, 2 out]
            n159 = case shown="Faux" w556 {
              tunnel: w557 -> [w565 _]
              tunnel: [w573 w583] -> w564
              tunnel: w563 -> [w573 w582]
              tunnel: [w571 w584] -> w562
              frame True {
                n160 = String Subset(string=w565, offset (0)=2) -> (substring=w570:string)  [unwired: 1 in]
                n161 = String Length(string=w570) -> (length=w568:i32)
                n162 = Multiply(x=0.5, y=w568) -> (x*y=w567:dbl)
                n163 = for {
                  N: w567 -> [_]
                  tunnel: w570 -> [w577]
                  tunnel: [w579] -> w569 mode=indexing
                  i -> [w576]
                  w575 = 2 ("length (rest)")
                  n164 = Multiply(x=w576, y=w575) -> (x*y=w574:i32)
                  n165 = String Subset(string=w577, offset (0)=w574, length (rest)=w575) -> (substring=w578:string)
                  n166 = Hexadecimal String To Number(string=w578, default (0uL)=u8 0 ("default (0 U32)")) -> (number=w579:u8)  [unwired: 1 in, 1 out]
                }
                n167 = Byte Array To String(unsigned byte array=w569) -> (string=w571:string)
              }
              frame False {
                n168 = Flatten To String(anything=waveform(dbl) {"t0"=timestamp(0 s since 1904-01-01), "dt"=0.0, "Y"=[]} ("Waveform 2"), error in (no error)=w582) -> (data string=w584:string, error out=w583:errorcluster)  [unwired: 2 in, 1 out]
              }
            }
          }
          frame "Timestamp" {
            n169 = Get Variant Attribute(Variant=w588, name=w586, default value (empty Variant)="") -> (found=w585:bool, value=w587:string)  [unwired: 1 in, 2 out]
            n170 = case shown="Faux" w585 {
              tunnel: w587 -> [w594 _]
              tunnel: [w602 w612] -> w593
              tunnel: w592 -> [w602 w611]
              tunnel: [w600 w613] -> w591
              frame True {
                n171 = String Subset(string=w594, offset (0)=2) -> (substring=w599:string)  [unwired: 1 in]
                n172 = String Length(string=w599) -> (length=w597:i32)
                n173 = Multiply(x=0.5, y=w597) -> (x*y=w596:dbl)
                n174 = for {
                  N: w596 -> [_]
                  tunnel: w599 -> [w606]
                  tunnel: [w608] -> w598 mode=indexing
                  i -> [w605]
                  w604 = 2 ("length (rest)")
                  n175 = Multiply(x=w605, y=w604) -> (x*y=w603:i32)
                  n176 = String Subset(string=w606, offset (0)=w603, length (rest)=w604) -> (substring=w607:string)
                  n177 = Hexadecimal String To Number(string=w607, default (0uL)=u8 0 ("default (0 U32)")) -> (number=w608:u8)  [unwired: 1 in, 1 out]
                }
                n178 = Byte Array To String(unsigned byte array=w598) -> (string=w600:string)
              }
              frame False {
                n179 = Flatten To String(anything=timestamp(0 s since 1904-01-01), error in (no error)=w611) -> (data string=w613:string, error out=w612:errorcluster)  [unwired: 2 in, 1 out]
              }
            }
          }
          frame "Digital Waveform" {
            n180 = Get Variant Attribute(Variant=w617, name=w614, default value (empty Variant)="") -> (found=w615:bool, value=w616:string)  [unwired: 1 in, 2 out]
            n181 = case shown="Faux" w615 {
              tunnel: w616 -> [w623 _]
              tunnel: [w631 w641] -> w622
              tunnel: w621 -> [w631 w640]
              tunnel: [w629 w642] -> w620
              frame True {
                n182 = String Subset(string=w623, offset (0)=2) -> (substring=w628:string)  [unwired: 1 in]
                n183 = String Length(string=w628) -> (length=w626:i32)
                n184 = Multiply(x=0.5, y=w626) -> (x*y=w625:dbl)
                n185 = for {
                  N: w625 -> [_]
                  tunnel: w628 -> [w635]
                  tunnel: [w637] -> w627 mode=indexing
                  i -> [w634]
                  w633 = 2 ("length (rest)")
                  n186 = Multiply(x=w634, y=w633) -> (x*y=w632:i32)
                  n187 = String Subset(string=w635, offset (0)=w632, length (rest)=w633) -> (substring=w636:string)
                  n188 = Hexadecimal String To Number(string=w636, default (0uL)=u8 0 ("default (0 U32)")) -> (number=w637:u8)  [unwired: 1 in, 1 out]
                }
                n189 = Byte Array To String(unsigned byte array=w627) -> (string=w629:string)
              }
              frame False {
                n190 = call <vilib>:"DWDT Empty Digital.vi"() -> ("digital waveform out"=w639:digitalwaveform)  [unwired: 5 in]
                n191 = Flatten To String(anything=w639, error in (no error)=w640) -> (data string=w642:string, error out=w641:errorcluster)  [unwired: 2 in, 1 out]
              }
            }
          }
          frame "Digital Data" {
            n192 = Get Variant Attribute(Variant=w645, name=w644, default value (empty Variant)="") -> (found=w643:bool, value=w646:string)  [unwired: 1 in, 2 out]
            n193 = case shown="Vrai" w643 {
              tunnel: w646 -> [w652 _]
              tunnel: [w660 w670] -> w651
              tunnel: w650 -> [w660 w669]
              tunnel: [w658 w671] -> w649
              frame True {
                n194 = String Subset(string=w652, offset (0)=2) -> (substring=w657:string)  [unwired: 1 in]
                n195 = String Length(string=w657) -> (length=w655:i32)
                n196 = Multiply(x=0.5, y=w655) -> (x*y=w654:dbl)
                n197 = for {
                  N: w654 -> [_]
                  tunnel: w657 -> [w664]
                  tunnel: [w666] -> w656 mode=indexing
                  i -> [w663]
                  w662 = 2 ("length (rest)")
                  n198 = Multiply(x=w663, y=w662) -> (x*y=w661:i32)
                  n199 = String Subset(string=w664, offset (0)=w661, length (rest)=w662) -> (substring=w665:string)
                  n200 = Hexadecimal String To Number(string=w665, default (0uL)=u8 0 ("default (0 U32)")) -> (number=w666:u8)  [unwired: 1 in, 1 out]
                }
                n201 = Byte Array To String(unsigned byte array=w656) -> (string=w658:string)
              }
              frame False {
                n202 = call <vilib>:"DTbl Empty Digital.vi"() -> ("digital data"=w668:digitaldata)  [unwired: 5 in]
                n203 = Flatten To String(anything=w668, error in (no error)=w669) -> (data string=w671:string, error out=w670:errorcluster)  [unwired: 2 in, 1 out]
              }
            }
          }
          frame "Array" {
            n204 = Get Variant Attribute(Variant=w675, name=w674, default value (empty Variant)="") -> (duplicate Variant=w672:variant, value=w673:string)  [unwired: 1 in, 2 out]
            n205 = call "Unprocess Array Elements.vi"("Variant Database"=w672, "Value"=w673, "Error In"=w680, "Name In"=w674, "Array Variant"=w678, "Queue In"=w682) -> ("Error Out"=w679:errorcluster, "Data Out"=w677:string, "Queue Out"=w681:refnum<queue>)  [unwired: 3 in]
          }
          frame Default {
            n206 = Get Variant Attribute(Variant=w686, name=w683, default value (empty Variant)="") -> (found=w684:bool, value=w685:string)  [unwired: 1 in, 2 out]
            n207 = case shown="Vrai" w684 {
              tunnel: w685 -> [w692 _]
              tunnel: [w700 w709] -> w691
              tunnel: w690 -> [w700 w710]
              tunnel: [w698 w711] -> w689
              frame True {
                n208 = String Subset(string=w692, offset (0)=2) -> (substring=w697:string)  [unwired: 1 in]
                n209 = String Length(string=w697) -> (length=w695:i32)
                n210 = Multiply(x=0.5, y=w695) -> (x*y=w693:dbl)
                n211 = for {
                  N: w693 -> [_]
                  tunnel: w697 -> [w704]
                  tunnel: [w706] -> w696 mode=indexing
                  i -> [w703]
                  w702 = 2 ("length (rest)")
                  n212 = Multiply(x=w703, y=w702) -> (x*y=w701:i32)
                  n213 = String Subset(string=w704, offset (0)=w701, length (rest)=w702) -> (substring=w705:string)
                  n214 = Hexadecimal String To Number(string=w705, default (0uL)=u8 0 ("default (0 U32)")) -> (number=w706:u8)  [unwired: 1 in, 1 out]
                }
                n215 = Byte Array To String(unsigned byte array=w696) -> (string=w698:string)
              }
              frame False {
                n216 = Flatten To String(anything="", error in (no error)=w710) -> (data string=w711:string, error out=w709:errorcluster)  [unwired: 2 in, 1 out]
              }
            }
          }
        }
        n217 = Get Queue Status(queue=w63, error in (no error)=w65) -> (queue out=w60:refnum<queue>, error out=w64:errorcluster, # elements in queue=w62:i32)  [unwired: 1 in, 5 out]
        n218 = Less Or Equal To 0?(x=w62) -> (x <= 0?=w61:bool)
      }
      n219 = Release Queue(queue=w29, error in (no error)=w31) -> (error out=w30:errorcluster)  [unwired: 1 in, 2 out]
      n220 = Concatenate Strings(w35) -> (w23:string)
      n221 = Flattened String To Variant(4:w30, 6:w23, 7:w38) -> (0:w37:errorcluster, 3:w36:variant)
    }
  }
  "Error Out" <- w13
  "Anything" <- w12
  "Found?" <- w9
